vi "WSP2_GetDateTimeStr.vi"() -> (1 "Time":string, 2 "error out":errorcluster)   [LabVIEW 2023]
uses:
  C:/Elatch-Bench-Test/VIs 64 bits/Elatch-Bench-Test/DLL/WSConnector.dll
  DLL/WSConnector.dll
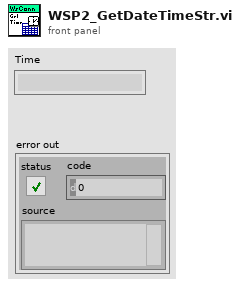
[diagram p1: front panel]
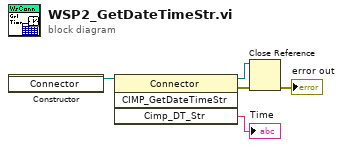
[diagram p0: block diagram]
diagram:
  n1 = constructor class="Connector"() -> (reference out=w5:refnum<k24>)  [unwired: 3 in, 2 out]
  n2 = invoke class="Connector" method="CIMP_GetDateTimeStr"(reference=w5) -> (reference out=w3:refnum<k24>, error out=w2:errorcluster, "Cimp_DT_Str"=→"Time":string)  [unwired: 3 in, 1 out]
  n3 = Close Reference(reference=w3, error in (no error)=w2) -> (error out=→"error out":errorcluster)
